vi "Rumble lister.vi"() -> ()   [LabVIEW 2023]
uses:
  <vilib>/Analysis/1siggen.llb/Ramp Pattern by Delta.vi
  <vilib>/httpClient/LabVIEWHTTPClient.lvlib
  <vilib>/ptbypt/NI_PtbyPt.lvlib
  <vilib>/Analysis/NI_AALBase.lvlib
panel:
  in  "private":bool
  in  "thumbs_dl":bool
  in  "thumbs":path caption="Thumbnails\nfolder"
  in  "scroll":bool=TRUE
  out "rate":bool caption="Rate limit"
  in  "Log file":path
  out "dt":dbl
  in  "Threads":i32=32 min=1
  out "Videos":string
  out "status":string
  in  "stop":bool
  in  "delay":u32 caption="Delay (ms)"
  in  "End ID":string="5bgshm"
  in  "Start ID":string="5bg000"
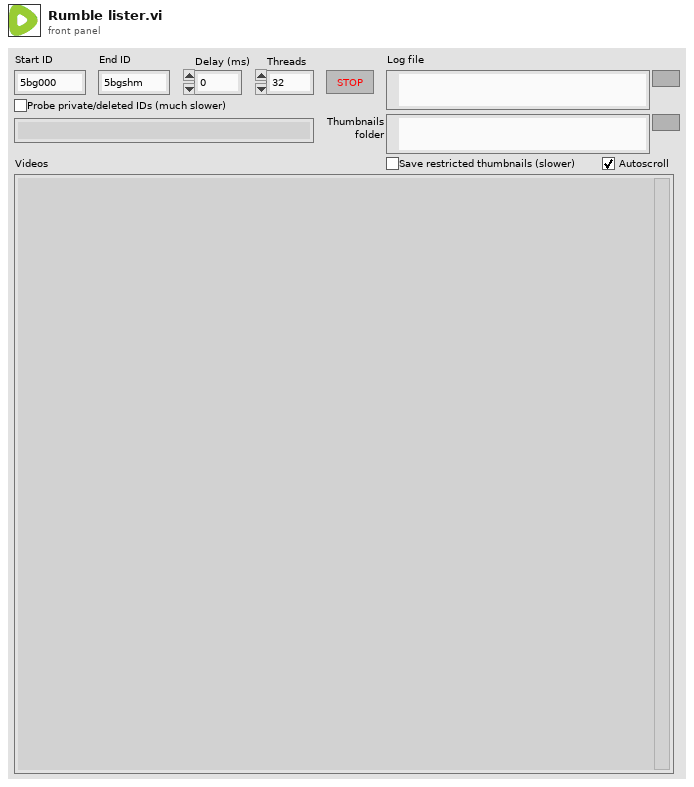
[diagram p1: front panel]
types:
  T1 = cluster{"URL":string, "Video info":string, "HTTP result":i32}
  T2 = enum16{"open", "replace", "create", "open or create", "replace or create", "replace or create with confirmation"}
  T3 = typedef "LabVIEWHTTPClient.lvlib/ClientHandle.ctl" = refnum<k1>
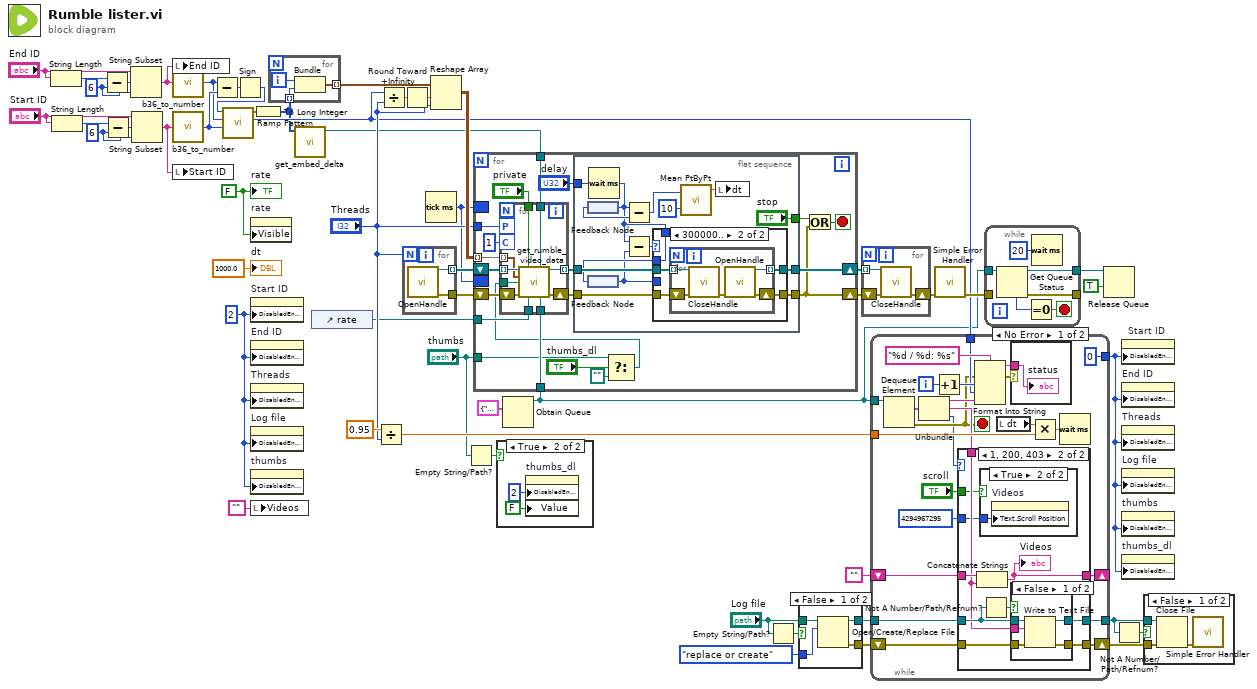
[diagram p0: block diagram]
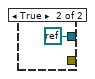
[diagram p4: hidden frame]
diagram:
  w10 = 6 ("y")
  w12 = 6 ("y")
  w21 = FALSE ("rate")
  w22 = u8 2
  n1 = String Length(string="End ID") -> (length=w8:i32)
  n2 = String Length(string="Start ID") -> (length=w15:i32)
  n3 = Subtract(x=w8, y=w10) -> (x-y=w9:i32)
  n4 = Subtract(x=w15, y=w12) -> (x-y=w13:i32)
  n5 = String Subset(string="End ID", offset (0)=w9, length (rest)=w10) -> (substring=w4:string)
  n6 = String Subset(string="Start ID", offset (0)=w13, length (rest)=w12) -> (substring=w5:string)
  n7 = local write "End ID"(w4) -> ()
  n8 = call "b36_to_number.vi"("Base36 string"=w4) -> ("Number"=w6:i32)
  n9 = call "b36_to_number.vi"("Base36 string"=w5) -> ("Number"=w11:i32)
  n10 = local write "Start ID"(w5) -> ()
  n11 = Subtract(x=w6, y=w11) -> (x-y=w25:i32)
  n12 = Sign(1:w25) -> (0:w19:i32)
  n13 = call-poly <vilib>:"Ramp Pattern.vi"("start"=w11, "end"=w6, "delta"=w19) -> ("samples"=w24:i32, "Ramp Pattern"=w26:dbl[])  [unwired: 6 in, 1 out]
  n14 = property on="rate" class="Bool (strict)"("Visible"=w21) -> ()  [unwired: 2 in, 2 out]
  n15 = property on="Start ID" class="Str"("DisabledEnum"=w22) -> ()  [unwired: 2 in, 2 out]
  n16 = property on="End ID" class="Str"("DisabledEnum"=w22) -> ()  [unwired: 2 in, 2 out]
  n17 = property on="Threads" class="DigNum (strict)"("DisabledEnum"=w22) -> ()  [unwired: 2 in, 2 out]
  n18 = property on="Log file" class="Path"("DisabledEnum"=w22) -> ()  [unwired: 2 in, 2 out]
  n19 = property on="thumbs" class="Path"("DisabledEnum"=w22) -> ()  [unwired: 2 in, 2 out]
  n20 = local write "Videos"("") -> ()
  n21 = To Long Integer(number=w26) -> (32bit integer=w2:i32[])
  n22 = for {
    tunnel: w2 -> [w55] mode=indexing
    tunnel: [w54] -> w3 mode=indexing
    i -> [w56]
    n23 = Bundle(w56, w55) -> (w54:cluster{i32, i32})  [unwired: 1 in]
  }
  n24 = call "get_embed_delta.vi"("Canonical IDs"=w2) -> ("Embed delta"=w1:refnum<queue>)  [unwired: 8 in, 2 out]
  n25 = control-ref of="rate"() -> (w29:refnum<vi>)
  n26 = Divide(x=0.95 ("y"), y="Threads") -> (x/y=w20:dbl)
  n27 = Divide(x=w24, y="Threads") -> (x/y=w48:dbl)
  n28 = Round Toward +Infinity(x=w48) -> (ceil(x): smallest int >= x=w47:dbl)
  n29 = for {
    N: "Threads" -> [_]
    tunnel: [w58] -> w53 mode=indexing
    tunnel: [w57] -> w52
    n30 = call <vilib>:"OpenHandle.vi"() -> ("client handle out"=w58:T3, "error out"=w57:errorcluster)  [unwired: 14 in]
  }
  n31 = Tick Count (ms)() -> (millisecond timer value=w31:u32)
  n32 = Reshape Array(w3, w47, "Threads") -> (w46:cluster{i32, i32}[][])
  n33 = Empty String/Path?(string/path="thumbs") -> (empty?=w16:bool)
  n34 = case shown="True" w16 {
    frame False {
    }
    frame True {
      n35 = property on="thumbs_dl" class="Bool (strict)"("DisabledEnum"=u8 2, "Value"=FALSE ("thumbs_dl")) -> ()  [unwired: 2 in, 2 out]
    }
  }
  n36 = Obtain Queue(element data type=T1 {"URL"="", "Video info"="", "HTTP result"=0} ("Result")) -> (queue out=w23:refnum<queue>)  [unwired: 4 in, 2 out]
  n37 = for {
    shift-right: [w73] -> w51
    shift-left: w53 -> [w77]
    shift-right: [w72] -> w50
    shift-left: w52 -> [w76]
    tunnel: w46 -> [w78] mode=indexing
    tunnel: "Threads" -> [w68]
    border: w31 -> [_]
    tunnel: w23 -> [w75]
    border: w31 -> [_]
    tunnel: w29 -> [w70]
    tunnel: "thumbs" -> [w66]
    tunnel: w1 -> [w61]
    stop <- w79 stop-if-true
    n38 = flat-sequence {
      tunnel: "delay" -> [w94]
      tunnel: w74 -> [w89]
      tunnel: w63 -> [w88]
      tunnel: [w87] -> w73
      tunnel: [w86] -> w72
      tunnel: ["stop"] -> w71
      frame #0 {
        n39 = feedback #1() -> (w93:u32)
        n40 = feedback #2() -> (w83:u32)
        n41 = Wait (ms)(milliseconds to wait=w94) -> (millisecond timer value=w85:u32)
        n42 = feedback-in #1(w85) -> ()
        n43 = Subtract(x=w85, y=w93) -> (x-y=w92:u32)
        n44 = Subtract(x=w85, y=w83) -> (x-y=w90:u32)
        n45 = case shown="300000.." w90 {
          tunnel: w89 -> [w97 w102]
          tunnel: w88 -> [w96 w101]
          tunnel: [w97 w100] -> w87
          tunnel: [w96 w99] -> w86
          tunnel: [w95 w98] -> w84
          tunnel: w85 -> [_ w98]
          tunnel: w83 -> [w95 _]
          frame Default {
          }
          frame 300000.. {
            n46 = for {
              tunnel: w102 -> [w107] mode=indexing
              shift-right: [w103] -> w99
              shift-left: w101 -> [w106]
              tunnel: [w104] -> w100 mode=indexing
              n47 = call <vilib>:"CloseHandle.vi"("client handle"=w107, "error in (no error)"=w106) -> ("error out"=w105:errorcluster)  [unwired: 13 in]
              n48 = call <vilib>:"OpenHandle.vi"("error in (no error)"=w105) -> ("client handle out"=w104:T3, "error out"=w103:errorcluster)  [unwired: 13 in]
            }
          }
        }
        n49 = feedback-in #2(w84) -> ()
        n50 = call <vilib>:"Mean PtByPt.vi"("x"=w92, "sample length"=10) -> ("mean"=w82:dbl)  [unwired: 2 in, 1 out]
        n51 = local write "dt"(w82) -> ()
      }
    }
    n52 = Select(t=w66, s="thumbs_dl", f=path "") -> (s? t:f=w64:path)
    n53 = for {
      tunnel: w78 -> [w116] mode=indexing
      tunnel: w77 -> [w117] mode=indexing
      tunnel: [w113] -> w74 mode=indexing
      tunnel: w75 -> [w112]
      tunnel: w70 -> [w114]
      workers-P: w68 -> [_]
      chunk-C: 1 -> [_]
      tunnel: w64 -> [w111]
      shift-right: [w110] -> w63
      shift-left: w76 -> [w115]
      tunnel: "private" -> [w109]
      tunnel: w61 -> [w108]
      n54 = call "get_rumble_video_data.vi"("HTTP client handle"=w117, "Private IDs (F)"=w109, "Embed delta"=w108, "Video ID"=w116, "Thumbnails folder"=w111, "error in (no error)"=w115, "Rate limit ref."=w114, "Result queue"=w112) -> ("client handle out"=w113:T3, "error out"=w110:errorcluster)  [unwired: 6 in]
    }
    n55 = Or(x=w71, y=w72) -> (x .or. y?=w79:bool)
  }
  n56 = Empty String/Path?(string/path="Log file") -> (empty?=w39:bool)
  n57 = case shown="False" w39 {
    tunnel: "Log file" -> [w120 _]
    tunnel: T2."replace or create" ("operation (0:open)") -> [w121 _]
    tunnel: [w119 refnum<k0> refnum] -> w36
    tunnel: [w118 _] -> w35
    frame False {
      n58 = Open/Create/Replace File(file path (use dialog)=w120, operation (0:open)=w121) -> (refnum out=w119:refnum<file>, error out=w118:errorcluster)  [unwired: 4 in, 1 out]
    }
    frame True {
    }
  }
  n59 = for {
    tunnel: w51 -> [w125] mode=indexing
    shift-right: [w123] -> w49
    shift-left: w50 -> [w124]
    n60 = call <vilib>:"CloseHandle.vi"("client handle"=w125, "error in (no error)"=w124) -> ("error out"=w123:errorcluster)  [unwired: 13 in]
  }
  n61 = while {
    shift-right: [w141] -> _
    shift-left: "" -> [w149]
    tunnel: w23 -> [w146]
    tunnel: w24 -> [w143]
    tunnel: w20 -> [w139]
    tunnel: w36 -> [w137]
    shift-right: [w135] -> w32
    shift-left: w35 -> [w136]
    tunnel: [w134] -> w33
    tunnel: [u8 0] -> w17
    i -> [w144]
    stop <- w129 stop-if-true
    n62 = Dequeue Element(queue=w146) -> (element=w145:T1, error out=w129:errorcluster)  [unwired: 2 in, 2 out]
    n63 = Unbundle(w145) -> ("URL"=w142:string, "Video info"=w132:string, "HTTP result"=w126:i32)
    n64 = Increment(x=w144) -> (x+1=w148:i32)
    n65 = case shown="1, 200, 403" w126 {
      tunnel: w149 -> [w153 w163]
      tunnel: [w153 w162] -> w141
      tunnel: w137 -> [w152 w161]
      tunnel: w136 -> [w151 w160]
      tunnel: [w151 w159] -> w135
      tunnel: [w152 w158] -> w134
      tunnel: w132 -> [_ w156]
      tunnel: "scroll" -> [_ w155]
      tunnel: u32 4294967295 ("Text.Scroll Position") -> [_ w154]
      frame Default {
      }
      frame 1, 200, 403 {
        n66 = Concatenate Strings(w163, w156) -> (w162:string)
        "Videos" <- w162
        n67 = case shown="True" w155 {
          tunnel: w154 -> [_ w164]
          frame False {
          }
          frame True {
            n68 = property on="Videos" class="Str"("Text.Scroll Position"=w164) -> ()  [unwired: 2 in, 2 out]
          }
        }
        n69 = Not A Number/Path/Refnum?(number/path/refnum=w161) -> (NaN/Path/Refnum?=w157:bool)
        n70 = case shown="False" w157 {
          tunnel: w156 -> [w169 _]
          tunnel: w161 -> [w168 w170]
          tunnel: w160 -> [w167 w171]
          tunnel: [w166 w171] -> w159
          tunnel: [w165 w170] -> w158
          frame False {
            n71 = Write to Text File(file (use dialog)=w168, text=w169, error in=w167) -> (refnum out=w165:refnum<file>, error out=w166:errorcluster)  [unwired: 1 in, 1 out]
          }
          frame True {
          }
        }
      }
    }
    n72 = Format Into String(format string="%d / %d: %s", error in=w129, w148, w143, w142) -> (resulting string=w131:string, error out=w130:errorcluster)  [unwired: 1 in]
    n73 = local read "dt"() -> (w140:dbl)
    n74 = case shown="No Error" w130 {
      tunnel: w131 -> [w150 _]
      frame No Error {
        "status" <- w150
      }
      frame Error {
      }
    }
    n75 = Multiply(x=w140, y=w139) -> (x*y=w138:dbl)
    n76 = Wait (ms)(milliseconds to wait=w138) -> ()  [unwired: 1 out]
  }
  n77 = call <vilib>:"Simple Error Handler.vi"("error in (no error)"=w49) -> ("error out"=w44:errorcluster)  [unwired: 4 in, 4 out]
  n78 = while {
    tunnel: w23 -> [w177]
    tunnel: w44 -> [_]
    tunnel: [w173] -> w43
    tunnel: [w172] -> _
    stop <- w175 stop-if-true
    n79 = Get Queue Status(queue=w177) -> (queue out=w173:refnum<queue>, error out=w172:errorcluster, # elements in queue=w176:i32)  [unwired: 2 in, 5 out]
    n80 = Equal To 0?(x=w176) -> (x = 0?=w175:bool)
    n81 = Wait (ms)(milliseconds to wait=u32 20) -> ()  [unwired: 1 out]
  }
  n82 = Release Queue(queue=w43, force destroy? (F)=TRUE) -> ()  [unwired: 1 in, 3 out]
  n83 = Not A Number/Path/Refnum?(number/path/refnum=w33) -> (NaN/Path/Refnum?=w34:bool)
  n84 = property on="Start ID" class="Str"("DisabledEnum"=w17) -> ()  [unwired: 2 in, 2 out]
  n85 = property on="End ID" class="Str"("DisabledEnum"=w17) -> ()  [unwired: 2 in, 2 out]
  n86 = property on="Threads" class="DigNum (strict)"("DisabledEnum"=w17) -> ()  [unwired: 2 in, 2 out]
  n87 = property on="Log file" class="Path"("DisabledEnum"=w17) -> ()  [unwired: 2 in, 2 out]
  n88 = property on="thumbs" class="Path"("DisabledEnum"=w17) -> ()  [unwired: 2 in, 2 out]
  n89 = property on="thumbs_dl" class="Bool (strict)"("DisabledEnum"=w17) -> ()  [unwired: 2 in, 2 out]
  n90 = case shown="False" w34 {
    tunnel: w33 -> [w179 _]
    tunnel: w32 -> [w180 _]
    frame False {
      n91 = Close File(refnum=w179, error in=w180) -> (error out=w178:errorcluster)  [unwired: 1 out]
      n92 = call <vilib>:"Simple Error Handler.vi"("error in (no error)"=w178) -> ()  [unwired: 4 in, 5 out]
    }
    frame True {
    }
  }
  "dt" <- 1000.0 ("dt")
  "rate" <- w21
